vi "Write Local Resource.vi"(8 "error in (no error)":errorcluster, 10 "Local Resource":refnum<k21>, 11 "4322 in":refnum<class "4322.lvclass">) -> (0 "error out":errorcluster, 3 "4322 out":refnum<class "4322.lvclass">)   [LabVIEW 2019, in "4322.lvlib" / "4322.lvclass"]
uses:
  Library/4322.lvclass
  Library/4322.lvclass/4322.ctl
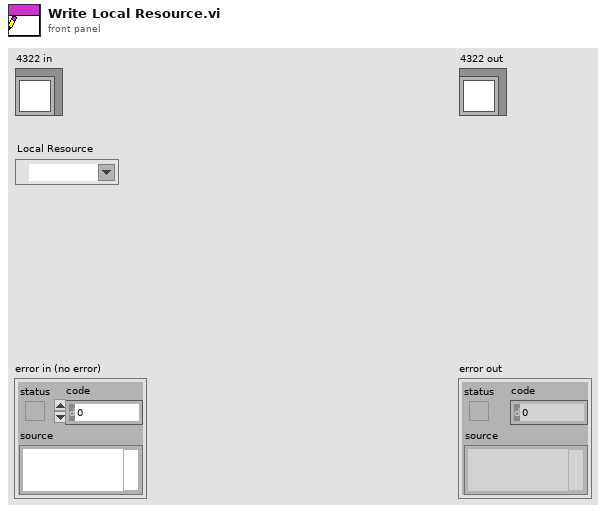
[diagram p1: front panel]
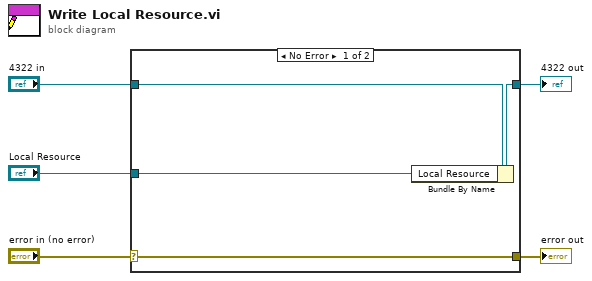
[diagram p0: block diagram]
diagram:
  n1 = case shown="No Error" "error in (no error)" {
    selector: "error in (no error)" -> [w9 w10]
    tunnel: [w9 w10] -> w4
    tunnel: [w7 w11] -> w2
    tunnel: "4322 in" -> [w8 w11]
    tunnel: "Local Resource" -> [w6 _]
    frame No Error {
      n2 = Bundle By Name(cluster=w8, "Local Resource"=w6) -> (w7:refnum<class "4322.lvclass">)
    }
    frame Error {
    }
  }
  "error out" <- w4
  "4322 out" <- w2
